vi "Hardware Parameters.vi"(7 "action":T2, 8 "error in":errorcluster, 11 "Hardware Parameters":T1={"Number Samples"=5000, "Time Between Points"=0.0, "Gain2 (dB)"=20, "CuttOff Freq1[MHz]"=9, "CuttOff Freq2[MHz]"=1, "Frequency"=8000000.0, "Phase"=180, "Power Level"=512, "Send Pulse"=FALSE, "Reset DDS"=FALSE, "TX CTRL"=FALSE, "RX CTRL"=FALSE, "Gain1 (dB)"=15, "Set DDS"=FALSE, "Start AQS"=FALSE, "Units"=0} {"Units" items=["us", "ms"]; "Gain1 (dB)" min=-5 max=45 step=1; "Power Level" max=1023 step=1; "Phase" max=270 step=90; "Frequency" min=1.0 format="%^#_6e"; "CuttOff Freq2[MHz]" min=1 max=30 step=1; "CuttOff Freq1[MHz]" min=1 max=30 step=1; "Gain2 (dB)" min=-5 max=45 step=1; "Time Between Points" min=0.0 step=1.0; "Number Samples" step=1}) -> (0 "error out":errorcluster, 3 "Hardware Paramentes out":T1={"Number Samples"=5000, "Time Between Points"=0.0, "Gain2 (dB)"=20, "CuttOff Freq1[MHz]"=9, "CuttOff Freq2[MHz]"=1, "Frequency"=8000000.0, "Phase"=180, "Power Level"=512, "Send Pulse"=FALSE, "Reset DDS"=FALSE, "TX CTRL"=FALSE, "RX CTRL"=FALSE, "Gain1 (dB)"=15, "Set DDS"=FALSE, "Start AQS"=FALSE, "Units"=0} {"Units" items=["us", "ms"]; "Gain1 (dB)" min=-5 max=45 step=1; "Power Level" max=1023 step=1; "Phase" max=270 step=90; "Frequency" min=1.0 format="%^#_6e"; "CuttOff Freq2[MHz]" min=1 max=30 step=1; "CuttOff Freq1[MHz]" min=1 max=30 step=1; "Gain2 (dB)" min=-5 max=45 step=1; "Time Between Points" min=0.0 step=1.0; "Number Samples" step=1})   [LabVIEW 2011]
uses:
  Hardware Parameters.ctl
  Controls/Hardware Control.ctl
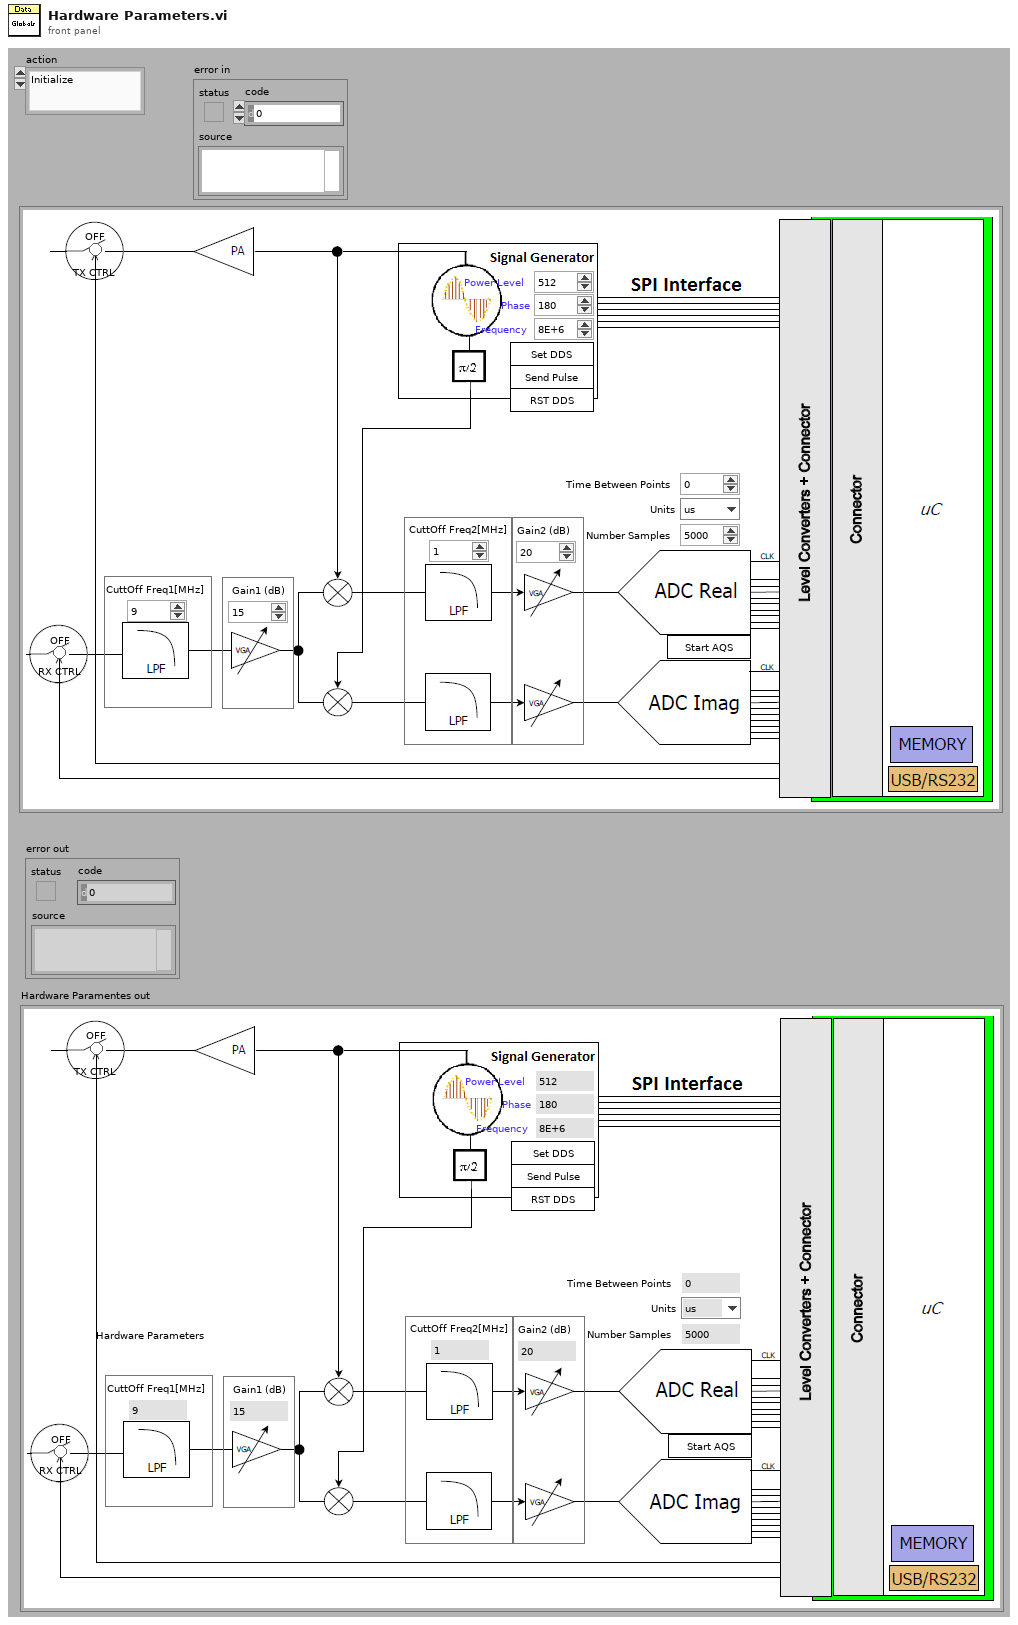
[diagram p1: front panel]
types:
  T1 = typedef "Hardware Control.ctl" = cluster{"Number Samples":u16, "Time Between Points":dbl, "Gain2 (dB)":i8, "CuttOff Freq1[MHz]":u8, "CuttOff Freq2[MHz]":u8, "Frequency":dbl, "Phase":u16, "Power Level":u16, "Send Pulse":bool, "Reset DDS":bool, "TX CTRL":bool, "RX CTRL":bool, "Gain1 (dB)":i8, "Set DDS":bool, "Start AQS":bool, "Units":u8}
  T2 = typedef "Hardware Parameters.ctl" = enum16{"Initialize", "Set Hardware Settings", "Get Hardware Settings", "Get Hardware CMD String"}
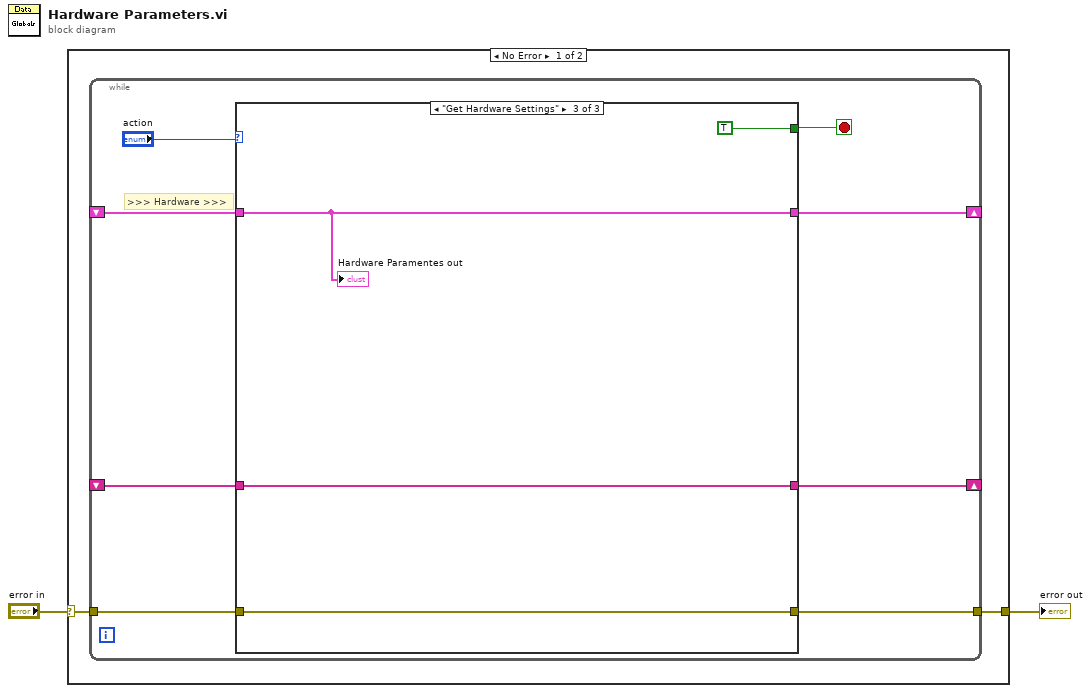
[diagram p0: block diagram]
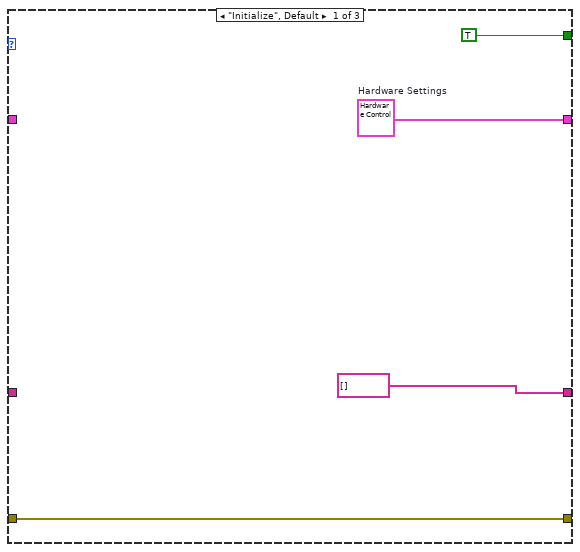
[diagram p2: hidden frame]
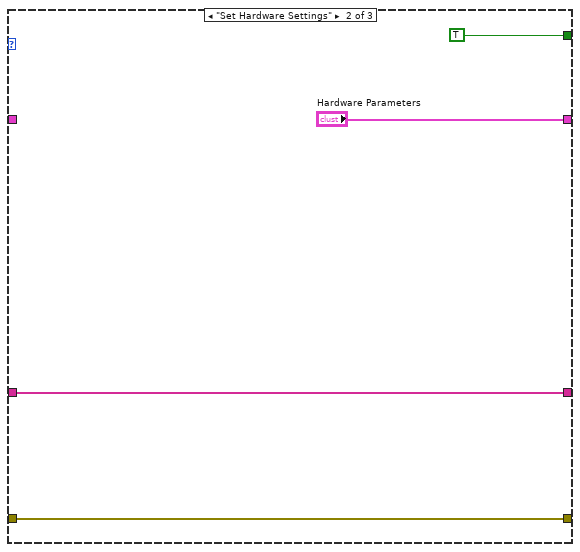
[diagram p3: hidden frame]
diagram:
  n1 = case shown="No Error" "error in" {
    selector: "error in" -> [w4 w25]
    tunnel: [w3 w25] -> w1
    frame No Error {
      n2 = while {
        tunnel: w4 -> [w12]
        tunnel: [w11] -> w3
        shift-right: [w9] -> _
        shift-left: _ -> [w8]
        shift-right: [w7] -> _
        shift-left: _ -> [w6]
        stop <- w10 stop-if-true
        # ">>> Hardware >>>"
        n3 = case shown="\"Get Hardware Settings\"" "action" {
          tunnel: w12 -> [w15 w20 w24]
          tunnel: [w15 w20 w24] -> w11
          tunnel: [TRUE TRUE TRUE] -> w10
          tunnel: [w13 "Hardware Parameters" w21] -> w9
          tunnel: w8 -> [_ _ w21]
          tunnel: [string[] [] w18 w22] -> w7
          tunnel: w6 -> [_ w18 w22]
          frame "Initialize", Default {
            w13 = T1 {"Number Samples"=0, "Time Between Points"=0.0, "Gain2 (dB)"=0, "CuttOff Freq1[MHz]"=0, "CuttOff Freq2[MHz]"=0, "Frequency"=0.0, "Phase"=0, "Power Level"=0, "Send Pulse"=FALSE, "Reset DDS"=FALSE, "TX CTRL"=FALSE, "RX CTRL"=FALSE, "Gain1 (dB)"=0, "Set DDS"=FALSE, "Start AQS"=FALSE, "Units"=0}  # Hardware Settings
          }
          frame "Set Hardware Settings" {
          }
          frame "Get Hardware Settings" {
            "Hardware Paramentes out" <- w21
          }
        }
      }
    }
    frame Error {
    }
  }
  "error out" <- w1
